vi "Get Force Units.vi"(8 "error in (no error)":errorcluster, 11 "ESM303 in":refnum<class "ESM303.lvclass">) -> (0 "error out":errorcluster, 2 "Force Units":T1=enum."N", 3 "ESM303 out":refnum<class "ESM303.lvclass">)   [LabVIEW 2018, in "ESM303.lvlib" / "ESM303.lvclass"]
uses:
  ESM303.lvclass
  builds/Force Test Stand/Force Test Stand/Force Test Stand.lvlibp/Custom Controls/Force Units.ctl
  builds/Force Test Stand/Force Test Stand/Force Test Stand.lvlibp/Force Test Stand.lvclass
  C:/Projects/LabVIEW/In-Progress/Jose Rivero-Diaz/builds/Force Test Stand/Force Test Stand/Force Test Stand.lvlibp/Force Test Stand.lvclass
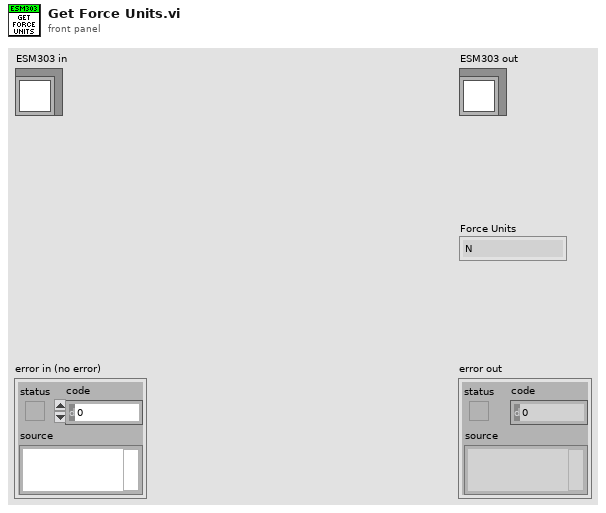
[diagram p1: front panel]
types:
  T1 = typedef "Force Test Stand.lvlibp/Force Test Stand.lvclass/Force Units.ctl" = enum16{"lbF", "ozF", "gF", "kgF", "N", "kN", "mN"}
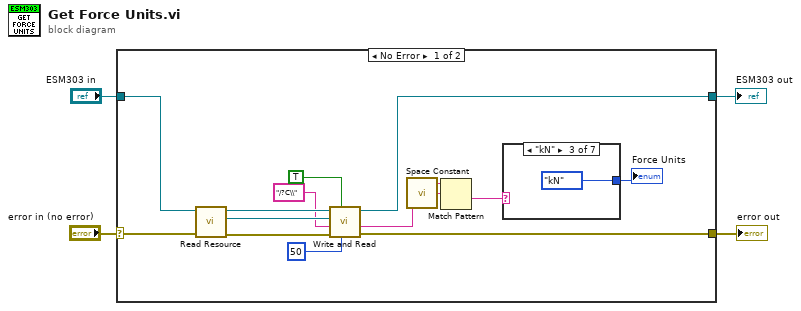
[diagram p0: block diagram]
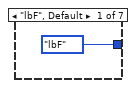
[diagram p2: hidden frame]
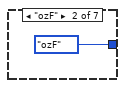
[diagram p3: hidden frame]
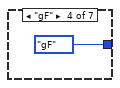
[diagram p4: hidden frame]
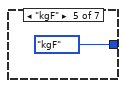
[diagram p5: hidden frame]
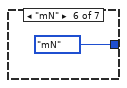
[diagram p6: hidden frame]
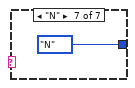
[diagram p7: hidden frame]
diagram:
  n1 = case shown="No Error" "error in (no error)" {
    selector: "error in (no error)" -> [w18 w27]
    tunnel: [w10 w27] -> w3
    tunnel: [w9 w26] -> w2
    tunnel: "ESM303 in" -> [w17 w26]
    frame No Error {
      n2 = call "Read Resource.vi"("error in (no error)"=w18, "Force Test Stand in"=w17) -> ("error out"=w16:errorcluster, "Resource"=w14:refnum<visa-resource-name>, "Force Test Stand out"=w15:refnum<class "ESM303.lvclass">)  [unwired: 7 in]
      n3 = call "Write and Read.vi"("Delay Before Read (ms)"=50, "Write & Read"=TRUE, "error in (no error)"=w16, "Command"="/?C\\", "VISA Refnum in"=w14, "ESM303 in"=w15) -> ("error out"=w10:errorcluster, "Response"=w7:string, "ESM303 out"=w9:refnum<class "ESM303.lvclass">)  [unwired: 3 in]
      n4 = call <vilib>:"Space Constant.vi"() -> ("String"=w6:string)
      n5 = Match Pattern(string=w7, regular expression=w6) -> (after substring=w5:string)  [unwired: 1 in, 3 out]
      n6 = case shown="\"kN\"" w5 {
        tunnel: [Force_Units."lbF" ("Force Units") Force_Units."ozF" ("Force Units") Force_Units."kN" ("Force Units") Force_Units."gF" ("Force Units") Force_Units."kgF" ("Force Units") Force_Units."mN" ("Force Units") Force_Units."N" ("Force Units")] -> w8
        frame "lbF", Default {
        }
        frame "ozF" {
        }
        frame "kN" {
        }
        frame "gF" {
        }
        frame "kgF" {
        }
        frame "mN" {
        }
        frame "N" {
        }
      }
      "Force Units" <- w8
    }
    frame Error {
    }
  }
  "error out" <- w3
  "ESM303 out" <- w2
